vi "Program25.vi"() -> ()   [LabVIEW 2020]
panel:
  in  "Kont.Numeryczna":i32
  in  "Kont.Logiczna":bool
  in  "Kont.Tekstowa":string
  out "Kont.Tekstowa 2":string
  out "Kont.Numeryczna 2":i32
  out "Logiczna 2":bool
  out "Tekstowa":string
  out "Numeryczna":i32
  out "Logiczna":bool
  out "Cluster 2":T1
  out "Cluster":T2
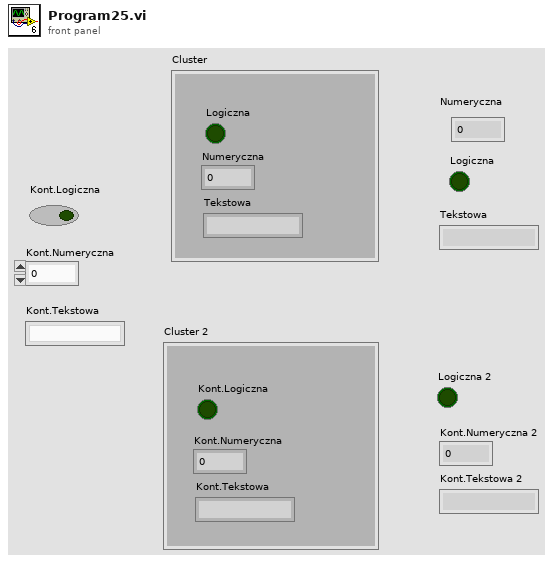
[diagram p1: front panel]
types:
  T1 = cluster{"Kont.Logiczna":bool, "Kont.Numeryczna":dbl, "Kont.Tekstowa":string}
  T2 = cluster{"Logiczna":bool, "Numeryczna":dbl, "Tekstowa":string}
  T3 = cluster{"Logiczna":bool, "Numeryczna":i32, "Tekstowa":string}
  T4 = cluster{"Kont.Logiczna":bool, "Kont.Numeryczna":i32, "Kont.Tekstowa":string}
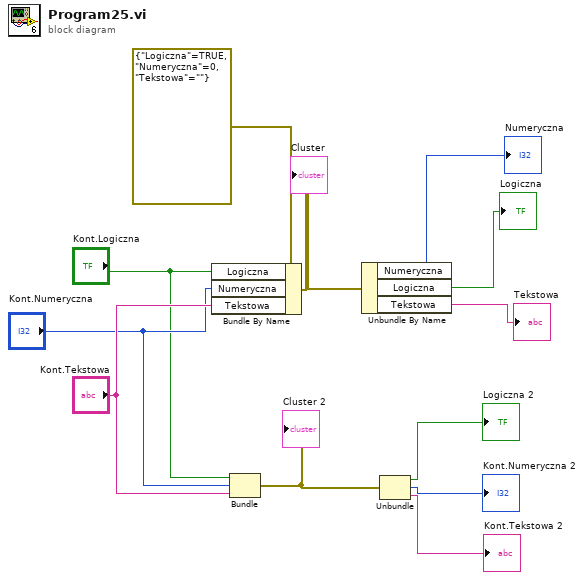
[diagram p0: block diagram]
diagram:
  n1 = Bundle By Name(cluster=T3 {"Logiczna"=TRUE, "Numeryczna"=0, "Tekstowa"=""}, "Logiczna"="Kont.Logiczna", "Numeryczna"="Kont.Numeryczna", "Tekstowa"="Kont.Tekstowa") -> (w12:T3)
  "Cluster" <- w12
  n2 = Bundle("Kont.Logiczna"="Kont.Logiczna", "Kont.Numeryczna"="Kont.Numeryczna", "Kont.Tekstowa"="Kont.Tekstowa") -> (w7:T4)  [unwired: 1 in]
  "Cluster 2" <- w7
  n3 = Unbundle By Name(w12) -> ("Numeryczna"=→"Numeryczna":i32, "Logiczna"=→"Logiczna":bool, "Tekstowa"=→"Tekstowa":string)
  n4 = Unbundle(w7) -> ("Kont.Logiczna"=→"Logiczna 2":bool, "Kont.Numeryczna"=→"Kont.Numeryczna 2":i32, "Kont.Tekstowa"=→"Kont.Tekstowa 2":string)
